vi "Create_Empty_Image_Greyscale.vi"(8 "error in (no error)":errorcluster, 10 "Preallocated Image Size (Default 0,0)":T1) -> (0 "error out":errorcluster, 3 "New Greyscale Image":refnum<data-value>)   [LabVIEW 2020, in "g_ar_toolkit.lvlib"]
uses:
  g_ar_toolkit.lvlib
  Image Size Cluster.ctl
  g_ar_toolkit.32.dll
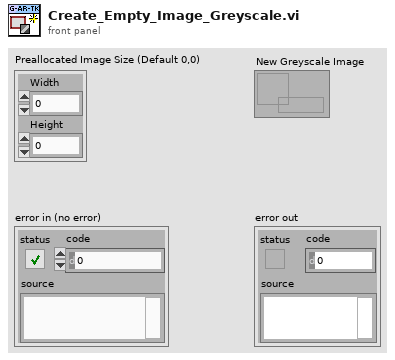
[diagram p1: front panel]
types:
  T1 = typedef "g_ar_toolkit.lvlib/Image Size Cluster.ctl" = cluster{"Width":u16, "Height":u16}
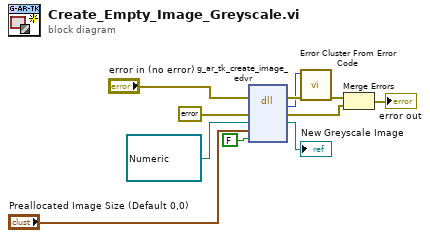
[diagram p0: block diagram]
diagram:
  n1 = dll-call lib="C:/serenial/libraries/g-augmented-reality-toolkit/LabVIEW/g_ar_toolkit/g_ar_toolkit.*.*" fn="g_ar_tk_create_image_edvr"(error in="error in (no error)", "error_cluster"=errorcluster {"status"=FALSE, "code"=0, "source"=""} ("error constant"), "EDVR"=refnum<data-value> refnum, "ImageSize"="Preallocated Image Size (Default 0,0)", "is_argb"=FALSE) -> (error out=w8:errorcluster, "MgErr"=w7:i32, "error_cluster"=w1:errorcluster, "EDVR"=→"New Greyscale Image":refnum<data-value>)  [unwired: 4 in, 1 out]
  n2 = call <vilib>:"Error Cluster From Error Code.vi"("error in (no error)"=w8, "error code (0)"=w7) -> ("error out"=w5:errorcluster)  [unwired: 7 in]
  n3 = Merge Errors(w5, w1) -> (→"error out":errorcluster)
